vi "Read configuration.vi"(8 "error in":errorcluster, 11 "DAQmx Watchdog editor node in":refnum<class "DAQmx Watchdog editor node.lvclass">) -> (0 "error out":errorcluster, 2 "configuration":refnum<class "NISE_CEF_serializable configuration.lvclass">, 3 "DAQmx Watchdog editor node out":refnum<class "DAQmx Watchdog editor node.lvclass">)   [LabVIEW 2014, in "DAQmx Watchdog editor node.lvclass"]
uses:
  DAQmx Watchdog editor node.lvclass
  <vilib>/NI/Configuration Framework/serializable configuration/NISE_CEF_serializable configuration.lvclass
  DAQmx Watchdog editor node.lvclass/DAQmx Watchdog editor node.ctl
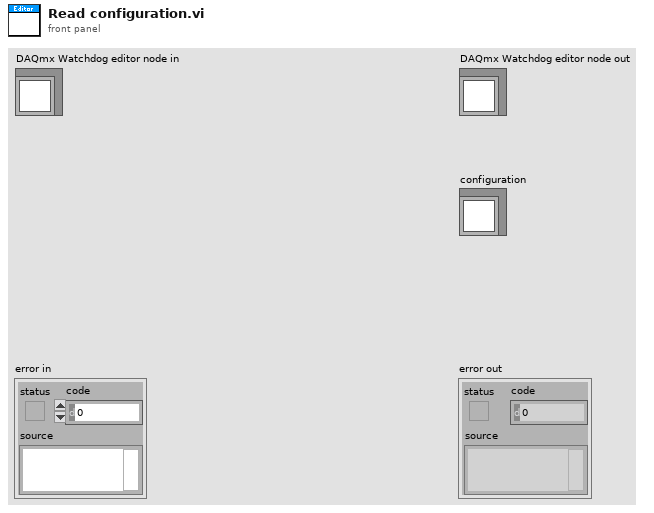
[diagram p1: front panel]
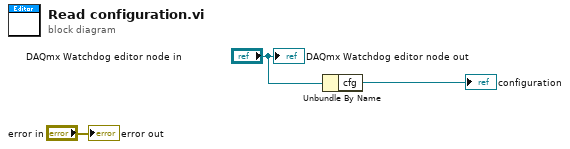
[diagram p0: block diagram]
diagram:
  n1 = Unbundle By Name("DAQmx Watchdog editor node in") -> ("cfg"=→"configuration":refnum<class "DAQmx Watchdog configuration.lvclass">)
  "error out" <- "error in"
  "DAQmx Watchdog editor node out" <- "DAQmx Watchdog editor node in"
